vi "CAL_GCP_L_EXT.vi"(0 "L_ROLL":sgl, 5 "ACC_Z":sgl, 9 "Param_In":T1) -> (4 "L_NUM":u32, 6 "L_Ctrl_Start":bool, 8 "L_RUN_OK":bool, 10 "L_GCP_EXT":sgl, 14 "L_GCP_Total_TIME":sgl, 15 "L_Period":u32)   [LabVIEW 2019]
uses:
  RT_GLOBAL.vi
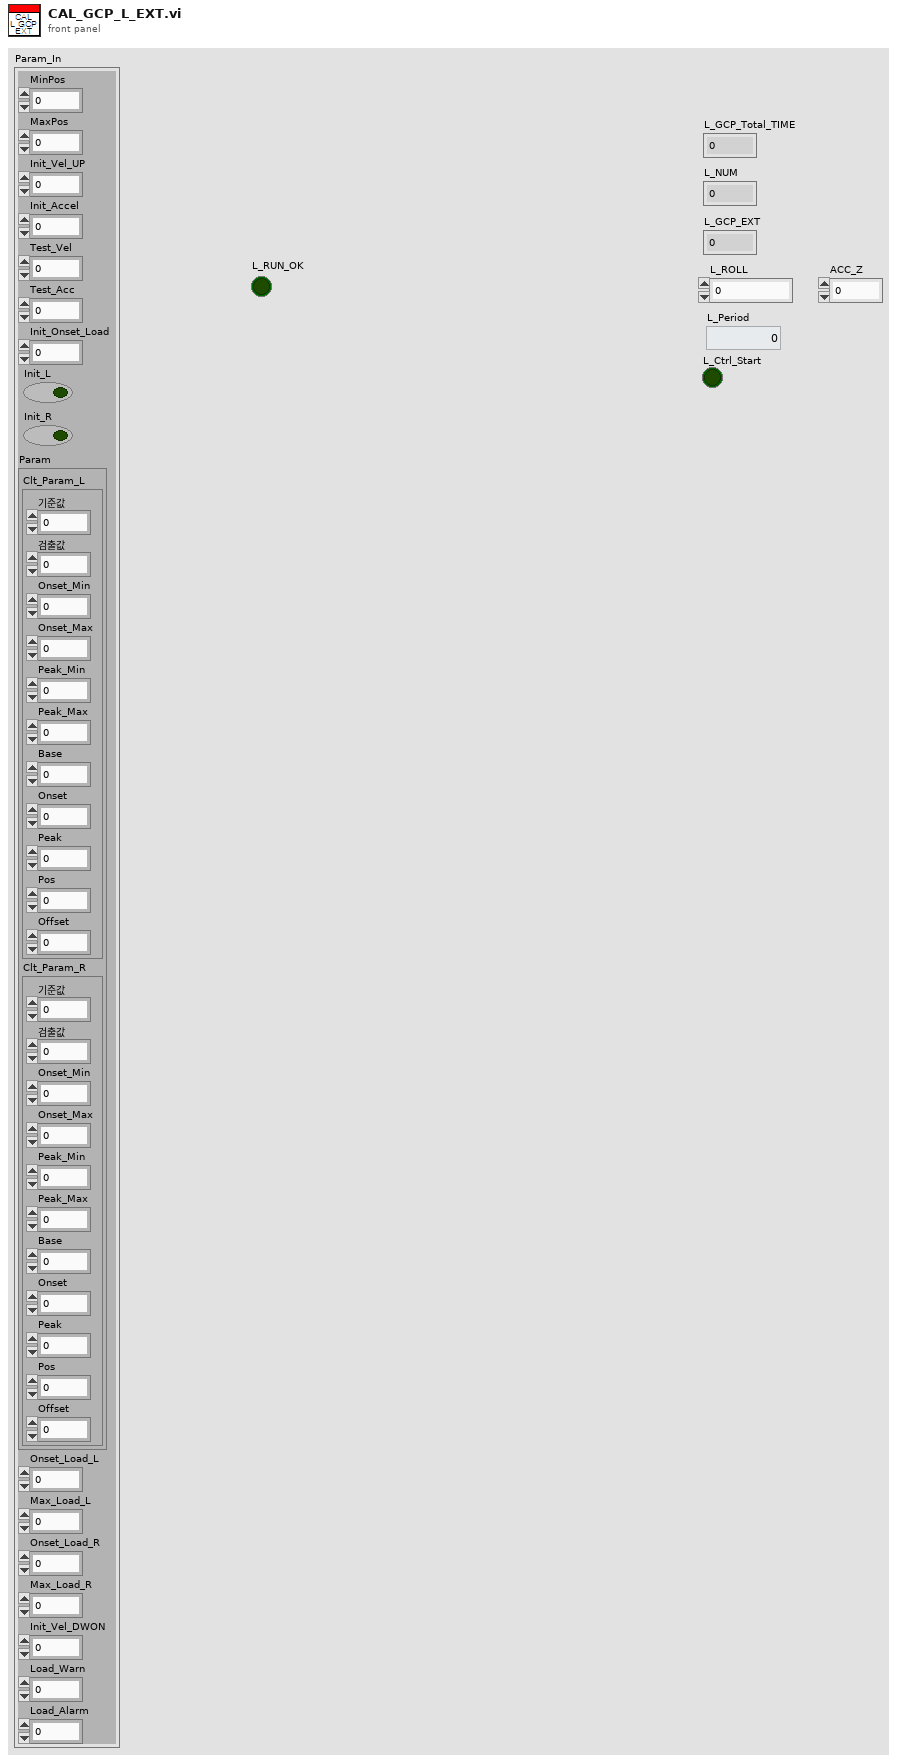
[diagram p1: front panel]
types:
  T1 = cluster{"MinPos":i32, "MaxPos":i32, "Init_Vel_UP":i32, "Init_Accel":u32, "Test_Vel":i32, "Test_Acc":u32, "Init_Onset_Load":sgl, "Init_L":bool, "Init_R":bool, "Param":cluster{"Clt_Param_L":cluster{"기준값":sgl, "검출값":sgl, "Onset_Min":sgl, "Onset_Max":sgl, "Peak_Min":sgl, "Peak_Max":sgl, "Base":i32, "Onset":i32, "Peak":i32, "Pos":i32, "Offset":sgl}, "Clt_Param_R":cluster{"기준값":sgl, "검출값":sgl, "Onset_Min":sgl, "Onset_Max":sgl, "Peak_Min":sgl, "Peak_Max":sgl, "Base":i32, "Onset":i32, "Peak":i32, "Pos":i32, "Offset":sgl}}, "Onset_Load_L":sgl, "Max_Load_L":sgl, "Onset_Load_R":sgl, "Max_Load_R":sgl, "Init_Vel_DWON":i32, "Load_Warn":sgl, "Load_Alarm":sgl}
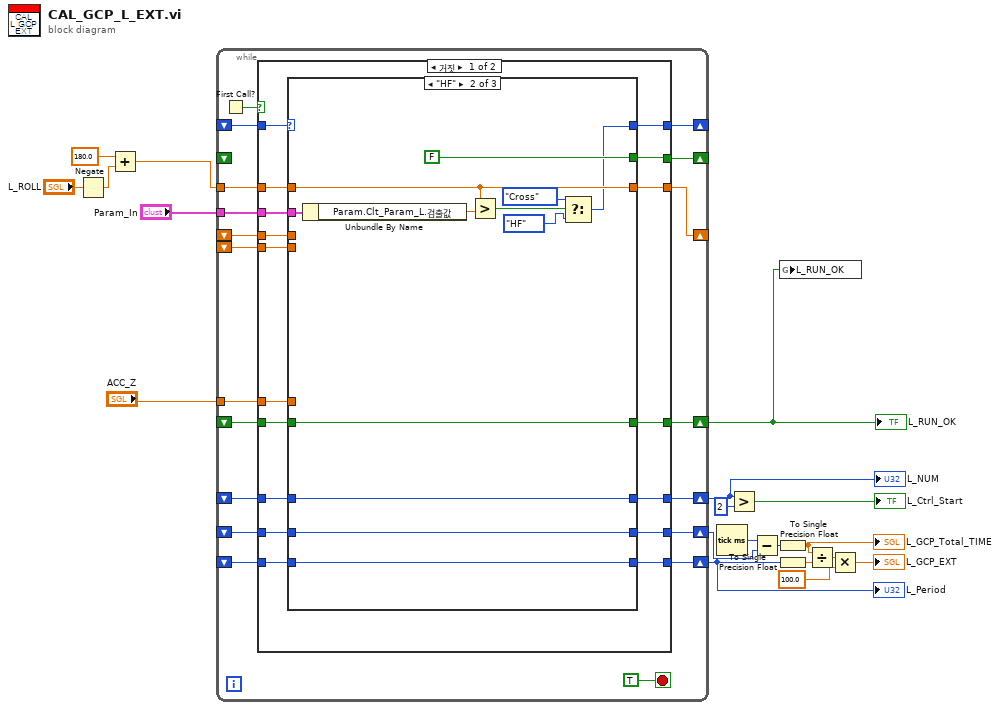
[diagram p0: block diagram]
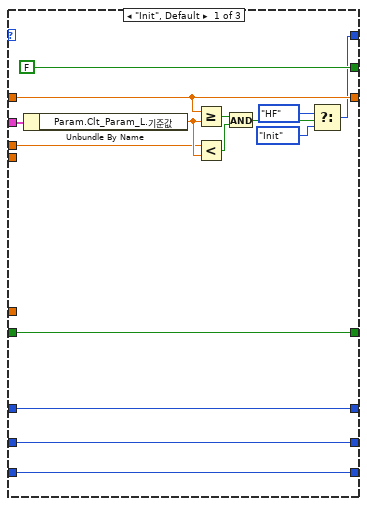
[diagram p2: hidden frame]
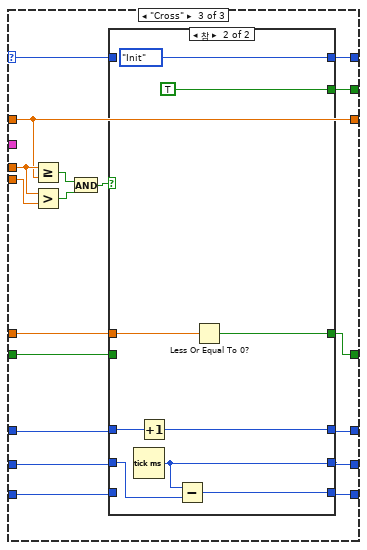
[diagram p3: hidden frame]
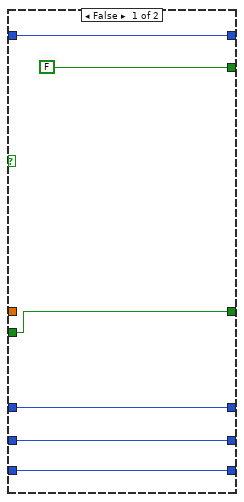
[diagram p4: hidden frame]
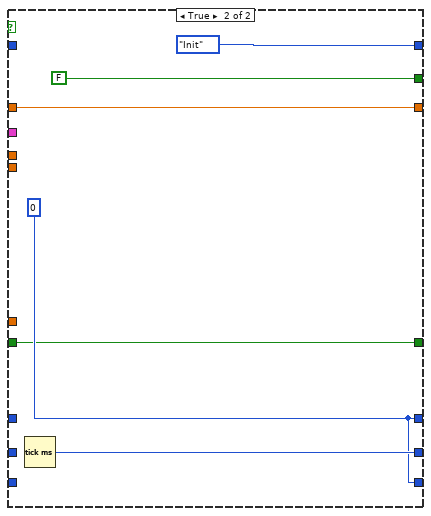
[diagram p5: hidden frame]
diagram:
  n1 = Negate(x="L_ROLL") -> (-x=w6:sgl)
  n2 = Add(x=sgl 180.0, y=w6) -> (x+y=w4:sgl)
  n3 = while {
    tunnel: w4 -> [w32]
    tunnel: "Param_In" -> [w25]
    shift-right: [w35] -> _
    shift-left: _ -> [w36]
    shift-right: [w34] -> _
    shift-left: _ -> [_]
    shift-right: [w33] -> _
    shift-left: _ -> [w24]
    shift-left: _ -> [w23]
    shift-right: [w30] -> w19
    shift-left: _ -> [w31]
    shift-right: [w29] -> w11
    shift-left: _ -> [w26]
    shift-right: [w28] -> w9
    shift-left: _ -> [w27]
    tunnel: "ACC_Z" -> [w22]
    shift-right: [w21] -> w1
    shift-left: _ -> [w20]
    stop <- TRUE stop-if-true
    n4 = First Call?() -> (First Call?: T/F=w37:bool)
    n5 = case shown="거짓" w37 {
      tunnel: w36 -> [w55 _]
      tunnel: [w50 enum16{"Init", "HF", "Cross"}."Init"] -> w35
      tunnel: [w51 FALSE] -> w34
      tunnel: [w52 w119] -> w33
      tunnel: w32 -> [w53 w119]
      tunnel: w31 -> [w48 _]
      tunnel: [w49 w117] -> w30
      tunnel: [w46 w118] -> w29
      tunnel: [w45 w117] -> w28
      tunnel: w27 -> [w44 _]
      tunnel: w26 -> [w47 _]
      tunnel: w25 -> [w54 _]
      tunnel: w24 -> [w43 _]
      tunnel: w23 -> [w42 _]
      tunnel: w22 -> [w41 _]
      tunnel: [w40 w116] -> w21
      tunnel: w20 -> [w39 w116]
      frame False {
        n6 = case shown="\"HF\"" w55 {
          selector: w55 -> [_ _ w100]
          tunnel: w54 -> [w63 w82 _]
          tunnel: w53 -> [w61 w77 w86]
          tunnel: [w61 w77 w86] -> w52
          tunnel: [FALSE FALSE w98] -> w51
          tunnel: [w60 w75 w99] -> w50
          tunnel: [w59 w74 w91] -> w49
          tunnel: w48 -> [w59 w74 w92]
          tunnel: w47 -> [w58 w73 w90]
          tunnel: [w58 w73 w88] -> w46
          tunnel: [w57 w72 w87] -> w45
          tunnel: w44 -> [w57 w72 w89]
          tunnel: w43 -> [w62 _ w97]
          tunnel: w42 -> [_ _ w96]
          tunnel: w41 -> [_ _ w85]
          tunnel: [w56 w71 w84] -> w40
          tunnel: w39 -> [w56 w71 w83]
          frame "Init", Default {
            n7 = Unbundle By Name(w63) -> ("Param.Clt_Param_L.기준값"=w64:sgl)
            n8 = Greater Or Equal?(x=w61, y=w64) -> (x >= y?=w69:bool)
            n9 = Less?(x=w62, y=w64) -> (x < y?=w68:bool)
            n10 = And(x=w69, y=w68) -> (x .and. y?=w67:bool)
            n11 = Select(t=enum16{"Init", "HF", "Cross"}."HF", s=w67, f=enum16{"Init", "HF", "Cross"}."Init") -> (s? t:f=w60:enum16{"Init", "HF", "Cross"})
          }
          frame "HF" {
            n12 = Unbundle By Name(w82) -> ("Param.Clt_Param_L.검출값"=w78:sgl)
            n13 = Greater?(x=w77, y=w78) -> (0:w79:bool)
            n14 = Select(t=enum16{"Init", "HF", "Cross"}."Cross", s=w79, f=enum16{"Init", "HF", "Cross"}."HF") -> (s? t:f=w75:enum16{"Init", "HF", "Cross"})
          }
          frame "Cross" {
            n15 = Greater Or Equal?(x=w97, y=w86) -> (x >= y?=w95:bool)
            n16 = Greater?(x=w97, y=w96) -> (0:w94:bool)
            n17 = And(x=w95, y=w94) -> (x .and. y?=w93:bool)
            n18 = case shown="참" w93 {
              tunnel: w100 -> [w102 _]
              tunnel: [w102 enum16{"Init", "HF", "Cross"}."Init"] -> w99
              tunnel: [FALSE TRUE] -> w98
              tunnel: w92 -> [w104 w113]
              tunnel: [w104 w112] -> w91
              tunnel: w90 -> [w105 w111]
              tunnel: w89 -> [w106 _]
              tunnel: [w106 w110] -> w87
              tunnel: [w105 w109] -> w88
              tunnel: w85 -> [_ w108]
              tunnel: [w101 w107] -> w84
              tunnel: w83 -> [w101 _]
              frame False {
              }
              frame True {
                n19 = Tick Count (ms)() -> (millisecond timer value=w109:u32)
                n20 = Increment(x=w113) -> (x+1=w112:u32)
                n21 = Subtract(x=w109, y=w111) -> (x-y=w110:u32)
                n22 = Less Or Equal To 0?(x=w108) -> (x <= 0?=w107:bool)
              }
            }
          }
        }
      }
      frame True {
        w117 = u32 0
        n23 = Tick Count (ms)() -> (millisecond timer value=w118:u32)
      }
    }
  }
  "L_NUM" <- w19
  "L_Period" <- w9
  "L_RUN_OK" <- w1
  n24 = Tick Count (ms)() -> (millisecond timer value=w13:u32)
  n25 = Greater?(x=w19, y=u32 2) -> (0:→"L_Ctrl_Start":bool)
  n26 = Subtract(x=w13, y=w11) -> (x-y=w12:u32)
  n27 = To Single Precision Float(number=w12) -> (single precision float=w8:sgl)
  "L_GCP_Total_TIME" <- w8
  n28 = To Single Precision Float(number=w9) -> (single precision float=w16:sgl)
  n29 = global write "RT_GLOBAL.vi" "L_RUN_OK"(w1) -> ()
  n30 = Divide(x=w8, y=w16) -> (x/y=w15:sgl)
  n31 = Multiply(x=w15, y=sgl 100.0) -> (x*y=→"L_GCP_EXT":sgl)
